vi "PWM Write.vi"(2 "error in (no error)":errorcluster, 3 "Ciclo de Trabajo":u8(knob) scale=0.0..255.0, 4 "VISA Refnum in":refnum<visa-resource-name>) -> (0 "error out":errorcluster, 1 "VISA Refnum out":refnum<visa-resource-name>)   [LabVIEW 2014]
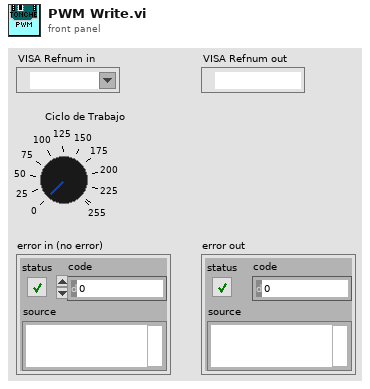
[diagram p1: front panel]
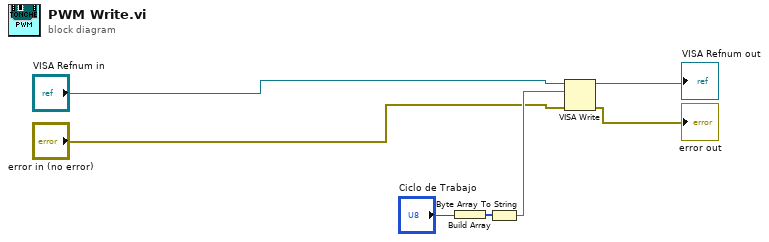
[diagram p0: block diagram]
diagram:
  n1 = Build Array("Ciclo de Trabajo") -> (w3:u8[])
  n2 = Byte Array To String(unsigned byte array=w3) -> (string=w4:string)
  n3 = VISA Write(VISA resource name="VISA Refnum in", write buffer=w4, error in (no error)="error in (no error)") -> (VISA resource name out=→"VISA Refnum out":refnum<visa-resource-name>, error out=→"error out":errorcluster)  [unwired: 1 out]
